vi "Write FIFO.vi"(10 "FIFO In":refnum<k21>="Tx Signal FPGA", 11 "Numeric":u32) -> ()   [LabVIEW 2017]
uses:
  <vilib>/rvi/Emulation/niFpgaSctlEmulationGetInTimedLoop.vi
  <vilib>/Utility/error.llb/Clear Errors.vi
  <vilib>/rvi/DataTransferAndStorage/Container/Common/niFpgaContainerExecOnDevCompGetState.vi
  <vilib>/rvi/Emulation/niFpgaEmulationIsFPGAContextNoSignature.vi
  <vilib>/rvi/errors/niFpgaSetErrorForExecOnDevCompSimple.vi
  <vilib>/rvi/eio/common/nirviEmuReportErrorAndStop.vi
  <vilib>/rvi/DataTransferAndStorage/Container/Common/niFpgaContainerGetUniqueNameForEmu.vi
  <vilib>/rvi/FIFO/Fifo_Resource/nirvififoEmulationSetSize.vi
  <vilib>/rvi/FIFO/Fifo_Resource/nirviFifoEmulationQueueMgr.vi
  <instcachedir>/0/nirviFifoEmulationQueueMgr_E5CAEC123FF24DC58D834DCA3CDAA9B5.lvgen/nirviFifoEmulationQueueMgr_E5CAEC123FF24DC58D834DCA3CDAA9B5_000.vi
  <vilib>/rvi/FIFO/Fifo_Resource/nirvififoEmulationDetermineInputValidOut.vi
  <vilib>/rvi/FIFO/Fifo_Resource/nirvififoEmulationCreateLock.vi
  <vilib>/rvi/Emulation/niFpgaProcessEmulError.vi
  <vilib>/rvi/FIFO/Fifo_Resource/nirvififoEmulationObtainLock.vi
  <vilib>/rvi/FIFO/Fifo_Resource/nirvififoEmulationReleaseLock.vi
  <vilib>/rvi/occurrence/nirviWaitOnOccurrenceBase.vi
  <vilib>/rvi/errors/nirviReportUnexpectedCaseInternalError.vi
  <vilib>/rvi/errors/nirviReportUnexpectedCaseInternalError (U32).vi
  <vilib>/rvi/interface/RandomDataEmulation/niFpgaRandomDataHandleErrors.vi
  <vilib>/rvi/DataTransferAndStorage/Container/XNode/niFpgaContainer.xnode
  <vilib>/rvi/FIFO/Fifo_Resource/niFpgaFifoEmulationRefIn.vi
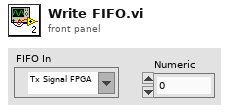
[diagram p1: front panel]
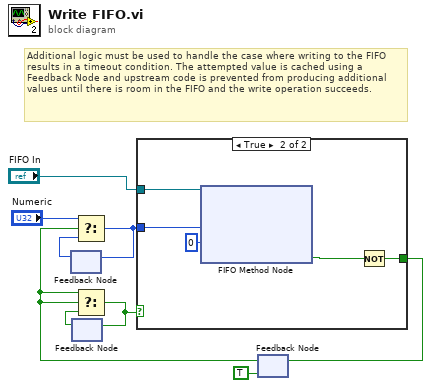
[diagram p0: block diagram]
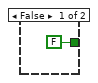
[diagram p2: hidden frame]
diagram:
  # "Additional logic must be used to handle the case where writing to the FIFO results in a timeout condition. The attempted value is cached using a Feedback Node and upstream code is prevented from producing additional values until there is room in the FIFO and the write operation succeeds."
  n1 = feedback #1() -> (w6:u32)  [unwired: 1 in]
  n2 = feedback #2() -> (w8:bool)  [unwired: 1 in]
  n3 = feedback #3(TRUE) -> (w3:bool)
  n4 = Select(t="Numeric", s=w3, f=w6) -> (s? t:f=w5:u32)
  n5 = feedback-in #1(w5) -> ()
  n6 = Select(t=w3, s=w3, f=w8) -> (s? t:f=w7:bool)
  n7 = feedback-in #2(w7) -> ()
  n8 = case shown="True" w7 {
    tunnel: w5 -> [_ w14]
    tunnel: [FALSE w12] -> w9
    tunnel: "FIFO In" -> [_ w11]
    frame False {
    }
    frame True {
      n9 = xnode ("FIFO Method Node")("Element"=w14, "Timeout"=0, "FIFO In"=w11) -> ("Timed Out?"=w13:bool)  [unwired: 1 out]
      n10 = Not(x=w13) -> (.not. x?=w12:bool)
    }
  }
  n11 = feedback-in #3(w9) -> ()
